vi "ProtoTracking_Distances.vi"() -> ()   [LabVIEW 2015]
uses:
  <vilib>/userdefined/High Color/IMAQdx.ctl
  <vilib>/Utility/file.llb/Read Delimited Spreadsheet (DBL).vi
  <vilib>/vision/driver/NI_Vision_Acquisition_Software.lvlib
  <vilib>/vision/NI_Vision_Development_Module.lvlib
  <userlib>/Newport ESP301/Newport ESP301.lvlib
panel:
  in  "Move":bool
  out "Image":T1(plugin-control)
  out "Centroid":cluster{"X Centroid":sgl, "Y Centroid":sgl} {"Y Centroid" format="%.2f"; "X Centroid" format="%.2f"}
  in  "Stop Button":bool
  in  "Camera Name":T2="cam0"
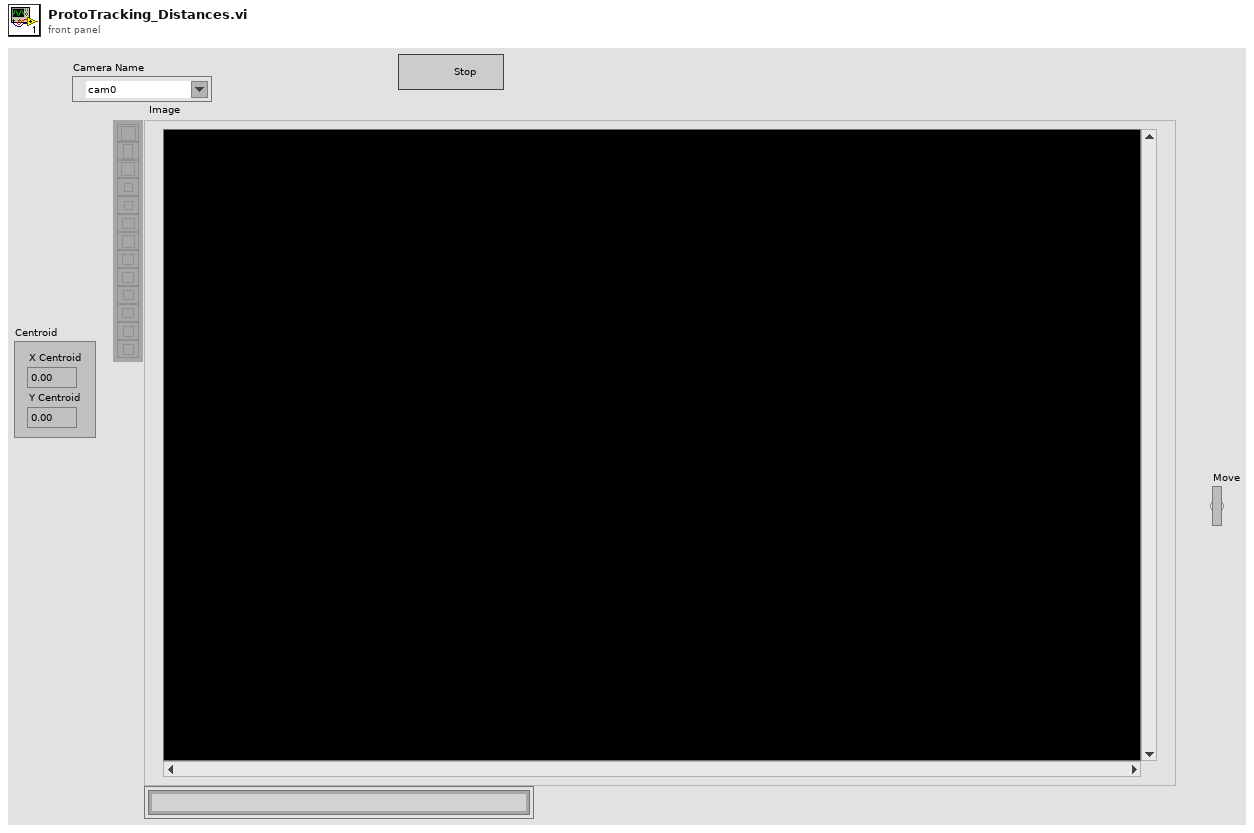
[diagram p1: front panel]
types:
  T1 = typedef "IMAQ Image.ctl" = refnum<image>
  T2 = typedef "IMAQdx.ctl" = refnum<k21>
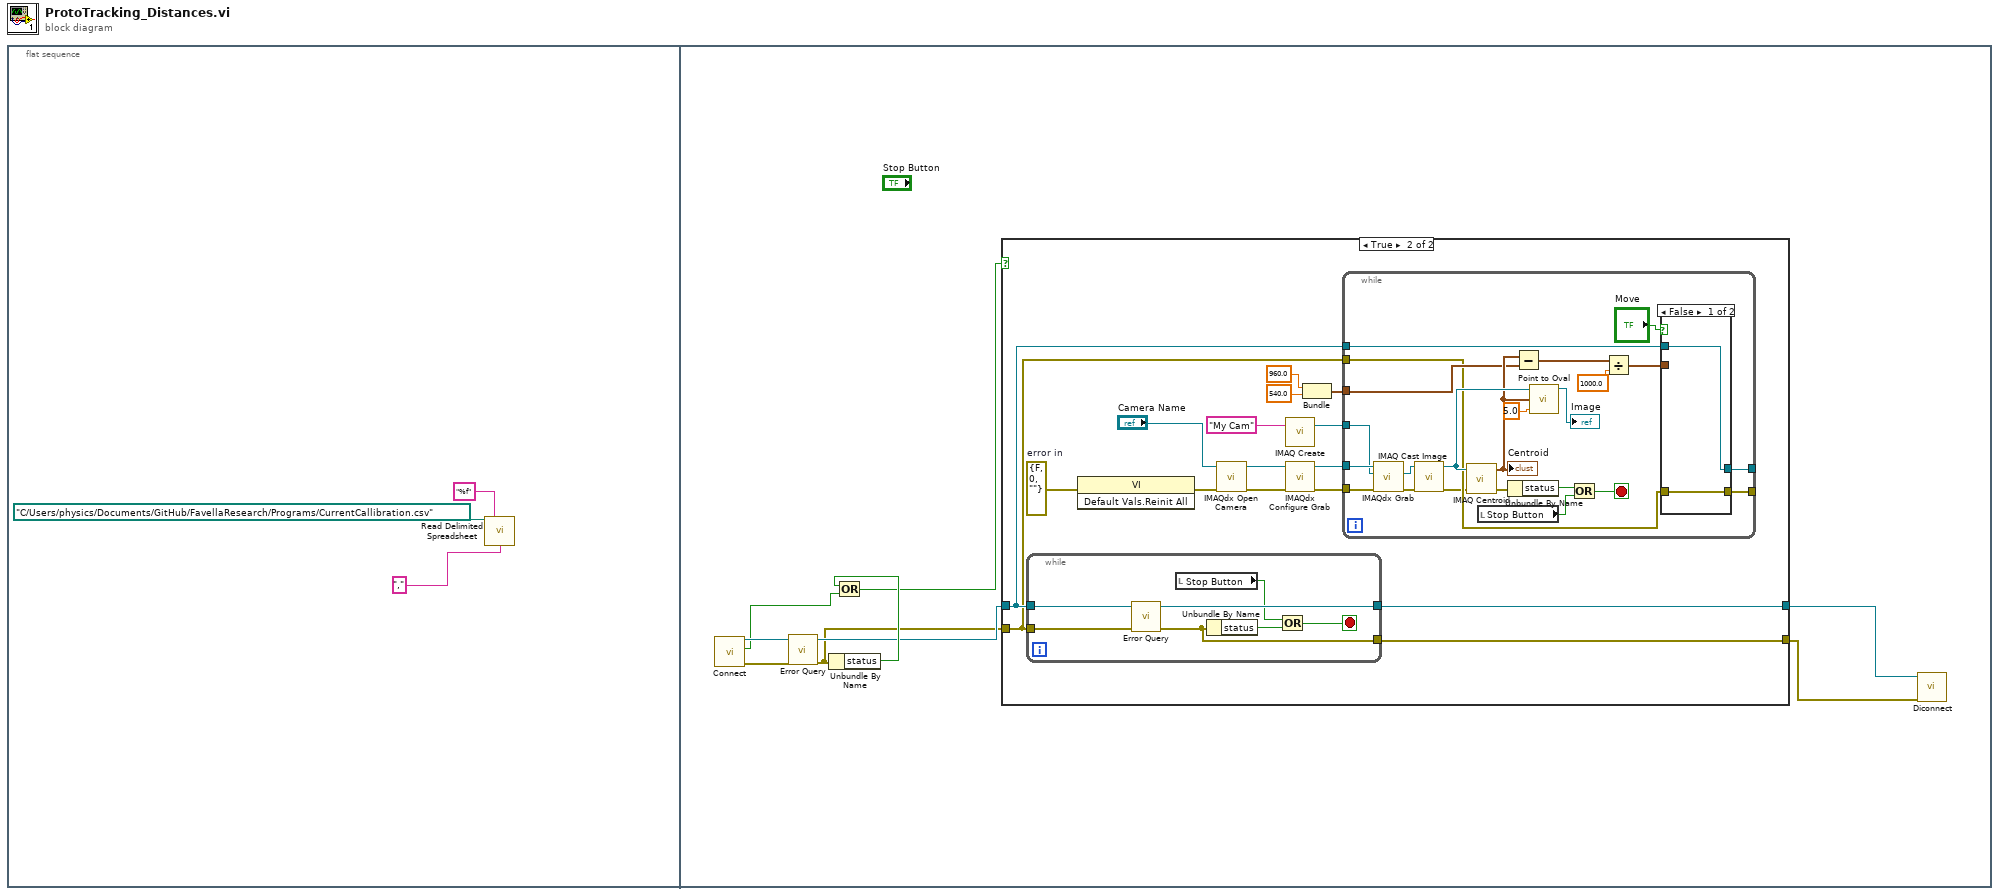
[diagram p0: block diagram]
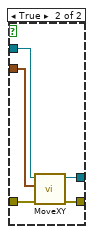
[diagram p3: hidden frame]
diagram:
  n1 = flat-sequence {
    frame #0 {
      n2 = call-poly <vilib>:"Read Delimited Spreadsheet.vi"("file path (dialog if empty)"=path "C:/Users/physics/Documents/GitHub/FavellaResearch/Programs/CurrentCallibration.csv", "format (%.3f)"="%f", "delimiter (\\t)"="," ("delimiter (\\t)")) -> ()  [unwired: 7 in, 6 out]
    }
    frame #1 {
      n3 = call "Connect.vi"() -> ("error out"=w9:errorcluster, "Connected"=w8:bool, "VISA resource name out"=w10:refnum<visa-resource-name>)  [unwired: 5 in]
      n4 = call <userlib>:"Error Query.vi"("error in (no error)"=w9, "VISA resource name"=w10) -> ("error out"=w4:errorcluster, "VISA resource name out"=w5:refnum<visa-resource-name>)  [unwired: 2 in, 2 out]
      n5 = Unbundle By Name(w4) -> ("status"=w7:bool)
      n6 = Or(x=w7, y=w8) -> (x .or. y?=w6:bool)
      n7 = case shown="True" w6 {
        tunnel: w5 -> [w13 w18]
        tunnel: w4 -> [w14 w17]
        tunnel: [w13 w16] -> w12
        tunnel: [w14 w15] -> w11
        frame False {
        }
        frame True {
          w29 = errorcluster {"status"=FALSE, "code"=0, "source"=""}  # error in
          n8 = while {
            tunnel: w18 -> [w37]
            tunnel: w17 -> [w36]
            tunnel: [w35] -> w16
            tunnel: [w34] -> w15
            stop <- w31 stop-if-true
            n9 = call <userlib>:"Error Query.vi"("error in (no error)"=w36, "VISA resource name"=w37) -> ("error out"=w34:errorcluster, "VISA resource name out"=w35:refnum<visa-resource-name>)  [unwired: 2 in, 2 out]
            n10 = local read "Stop Button"() -> (w33:bool)
            n11 = Unbundle By Name(w34) -> ("status"=w32:bool)
            n12 = Or(x=w33, y=w32) -> (x .or. y?=w31:bool)
          }
          n13 = invoke class="VI" method="Default Vals.Reinit All"(error in=w29) -> (error out=w28:errorcluster)  [unwired: 2 in, 2 out]
          n14 = call <vilib>:"IMAQdx Open Camera.vi"("error in"=w28, "Session In"="Camera Name") -> ("error out"=w25:errorcluster, "Session Out"=w26:T2)  [unwired: 8 in]
          n15 = call "IMAQ Create"("Image Name"="My Cam") -> ("New Image"=w23:T1)  [unwired: 4 in, 1 out]
          n16 = call <vilib>:"IMAQdx Configure Grab.vi"("error in"=w25, "Session In"=w26) -> ("error out"=w22:errorcluster, "Session Out"=w24:T2)  [unwired: 8 in]
          n17 = Bundle(960.0, 540.0) -> (w19:cluster{dbl, dbl})  [unwired: 1 in]
          n18 = while {
            tunnel: w24 -> [w60]
            tunnel: w23 -> [w59]
            tunnel: w22 -> [w58]
            tunnel: w18 -> [w42]
            tunnel: w17 -> [w41]
            tunnel: [w44] -> _
            tunnel: [w43] -> _
            tunnel: w19 -> [w47]
            stop <- w55 stop-if-true
            n19 = call <vilib>:"IMAQdx Grab.vi"("error in"=w58, "Image In"=w59, "Session In"=w60) -> ("error out"=w52:errorcluster, "Image Out"=w53:T1)  [unwired: 5 in, 2 out]
            n20 = call "IMAQ Cast Image"("error in (no error)"=w52, "Image Src"=w53) -> ("error out"=w38:errorcluster, "Image Dst Out"=w49:T1)  [unwired: 8 in]
            n21 = call "IMAQ Centroid"("error in (no error)"=w38, "Image"=w49) -> ("error out"=w54:errorcluster, "Centroid"=w48:cluster{"X Centroid":sgl, "Y Centroid":sgl})  [unwired: 2 in]
            "Centroid" <- w48
            n22 = local read "Stop Button"() -> (w56:bool)
            n23 = Unbundle By Name(w54) -> ("status"=w57:bool)
            n24 = Subtract(x=w48, y=w47) -> (x-y=w46:cluster{dbl, dbl})
            n25 = call "Point to Oval.vi"("Image In"=w49, "Point"=w48, "Size"=5.0) -> ("Image Out"=→"Image":T1)  [unwired: 3 in]
            n26 = Or(x=w57, y=w56) -> (x .or. y?=w55:bool)
            n27 = Divide(x=w46, y=1000.0) -> (x/y=w40:cluster{dbl, dbl})
            n28 = case shown="False" "Move" {
              tunnel: [w62 w67] -> w44
              tunnel: [w61 w66] -> w43
              tunnel: w42 -> [w62 w65]
              tunnel: w41 -> [w61 w64]
              tunnel: w40 -> [_ w63]
              frame False {
              }
              frame True {
                n29 = call "MoveXY.vi"("error in (no error)"=w64, "XY Cluster"=w63, "VISA resource name"=w65) -> ("error out"=w66:errorcluster, "VISA resource Out"=w67:refnum<visa-resource-name>)  [unwired: 7 in]
              }
            }
          }
        }
      }
      n30 = call "Diconnect.vi"("error in (no error)"=w11, "VISA resource name"=w12) -> ()  [unwired: 6 in]
    }
  }
